vi "eventForceActuatorInfo.vi"(8 "error in (no error)":errorcluster, 11 "Publisher in":refnum<class "Publisher.lvclass">) -> (0 "error out":errorcluster, 3 "Publisher out":refnum<class "Publisher.lvclass">)   [LabVIEW 2016, in "Publisher.lvclass"]
uses:
  Publisher.lvclass
  Publisher.lvclass/Publisher.ctl
  Communicator/M1M3SAL/M1M3SAL.lvclass/M1M3SAL.ctl
  Communicator/M1M3SAL/writeHeader.vi
  Communicator/M1M3SAL/writeDBL.vi
  Communicator/M1M3SAL/writeI32Array.vi
  Communicator/M1M3SAL/writeSGLArray.vi
  Communicator/M1M3SAL/writeI64Array.vi
  Communicator/M1M3SAL/writeU8Array.vi
  Communicator/M1M3SAL/writeBooleanArray.vi
  Communicator/M1M3SAL/writeI32.vi
  Communicator/M1M3SAL/writeU8.vi
  Communicator/M1M3SAL/writeSGL.vi
  Communicator/M1M3SAL/writeI64.vi
  Communicator/M1M3SAL/writeBoolean.vi
  Communicator/M1M3SAL/M1M3SAL.lvclass
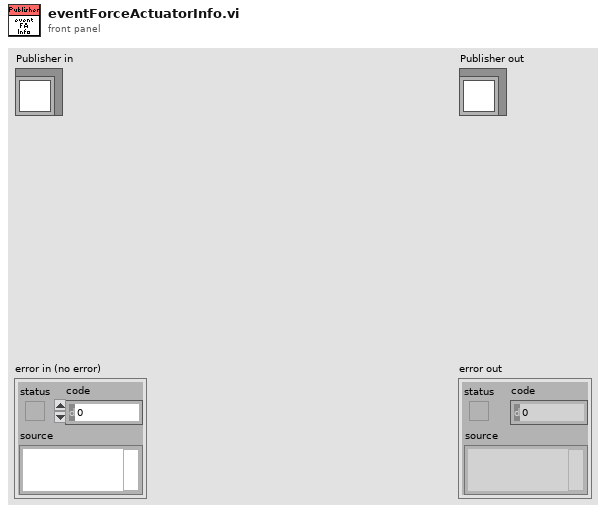
[diagram p1: front panel]
types:
  T1 = typedef "M1M3SupportTopics.lvlib/EventForceActuatorInfo.ctl" = cluster{"Timestamp":T2, "ReferenceId":i32[], "XPosition":sgl[], "YPosition":sgl[], "ZPosition":sgl[], "ILCUniqueId":i64[], "ILCApplicationType":u8[], "NetworkNodeType":u8[], "ILCSelectedOptions":u8[], "NetworkNodeOptions":u8[], "MajorRevision":u8[], "MinorRevision":u8[], "ADCScanRate":u8[], "MainADCCalibrationK1":sgl[], "MainADCCalibrationK2":sgl[], "MainADCCalibrationK3":sgl[], "MainADCCalibrationK4":sgl[], "MainAxialLoadCellOffset":sgl[], "MainLateralLoadCellOffset":sgl[], "MainAxialLoadCellSensitivity":sgl[], "MainLateralLoadCellSensitivity":sgl[], "BackupADCCalibrationK1":sgl[], "BackupADCCalibrationK2":sgl[], "BackupADCCalibrationK3":sgl[], "BackupADCCalibrationK4":sgl[], "BackupAxialLoadCellOffset":sgl[], "BackupLateralLoadCellOffset":sgl[], "BackupAxialLoadCellSensitivity":sgl[], "BackupLateralLoadCellSensitivity":sgl[], "DCAAxialGain":sgl[], "DCALateralGain":sgl[], "DCAUniqueId":i64[], "DCAFirmwareType":u8[], "DCAMajorRevision":u8[], "DCAMinorRevision":u8[], "MainCalibrationError":bool[], "BackupCalibrationError":bool[], "DCAFirmwareUpdate":bool[], "UniqueIdCRCError":bool[], "ApplicationTypeMismatch":bool[], "ApplicationMissing":bool[], "ApplicationCRCMismatch":bool[], "OneWireMissing":bool[], "OneWire1Mismatch":bool[], "OneWire2Mismatch":bool[], "DCAUniqueIdCRCError":bool[], "DCAMainCalibrationError":bool[], "DCABackupCalibrationError":bool[], "DCAApplicationMissing":bool[], "DCAApplicationCRCMismatch":bool[], "DCABootloaderActive":bool[]}
  T2 = typedef "M1M3SupportTopics.lvlib/Timestamp.ctl" = dbl
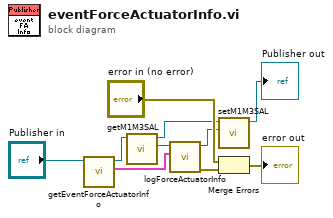
[diagram p0: block diagram]
diagram:
  n1 = call "getEventForceActuatorInfo.vi"("Publisher in"="Publisher in") -> ("EventForceActuatorInfo"=w3:T1, "Publisher out"=w7:refnum<class "Publisher.lvclass">)  [unwired: 9 in]
  n2 = call "getM1M3SAL.vi"("Publisher in"=w7) -> ("M1M3SAL"=w4:refnum<class "M1M3SAL.lvclass">, "Publisher out"=w6:refnum<class "Publisher.lvclass">)  [unwired: 9 in]
  n3 = call "logForceActuatorInfo.vi"("EventForceActuatorInfo"=w3, "M1M3SAL in"=w4) -> ("error out"=w1:errorcluster, "M1M3SAL out"=w2:refnum<class "M1M3SAL.lvclass">)  [unwired: 8 in]
  n4 = call "setM1M3SAL.vi"("M1M3SAL"=w2, "Publisher in"=w6) -> ("Publisher out"=→"Publisher out":refnum<class "Publisher.lvclass">)  [unwired: 9 in]
  n5 = Merge Errors("error in (no error)", w1) -> (→"error out":errorcluster)
